vi "退出所有.vi"() -> ()   [LabVIEW 2013]
panel:
  in  "退出所有":bool
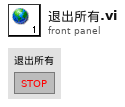
[diagram p1: front panel]
diagram:
